vi "Page_Advanced_WriteAll.vi"(6 "ctl references":T1, 8 "error in (no error)":errorcluster, 11 "AB_Application in":refnum<class "AB_Application.lvclass">) -> (0 "error out":errorcluster, 3 "AB_Application out":refnum<class "AB_Application.lvclass">)   [LabVIEW 2020, in "AB_Application.lvclass"]
uses:
  <vilib>/AppBuilder/AB_Classes/Application/AB_Application.lvclass
  <vilib>/AppBuilder/AB_Classes/Application/AB_Application.lvclass/AB_Application.ctl
  <vilib>/AppBuilder/AB_Classes/TargetFile/AB_Targetfile.lvclass
  <resource>/Framework/Providers/Builds/AppBuilder/AB_UI_Page_Advanced_References.ctl
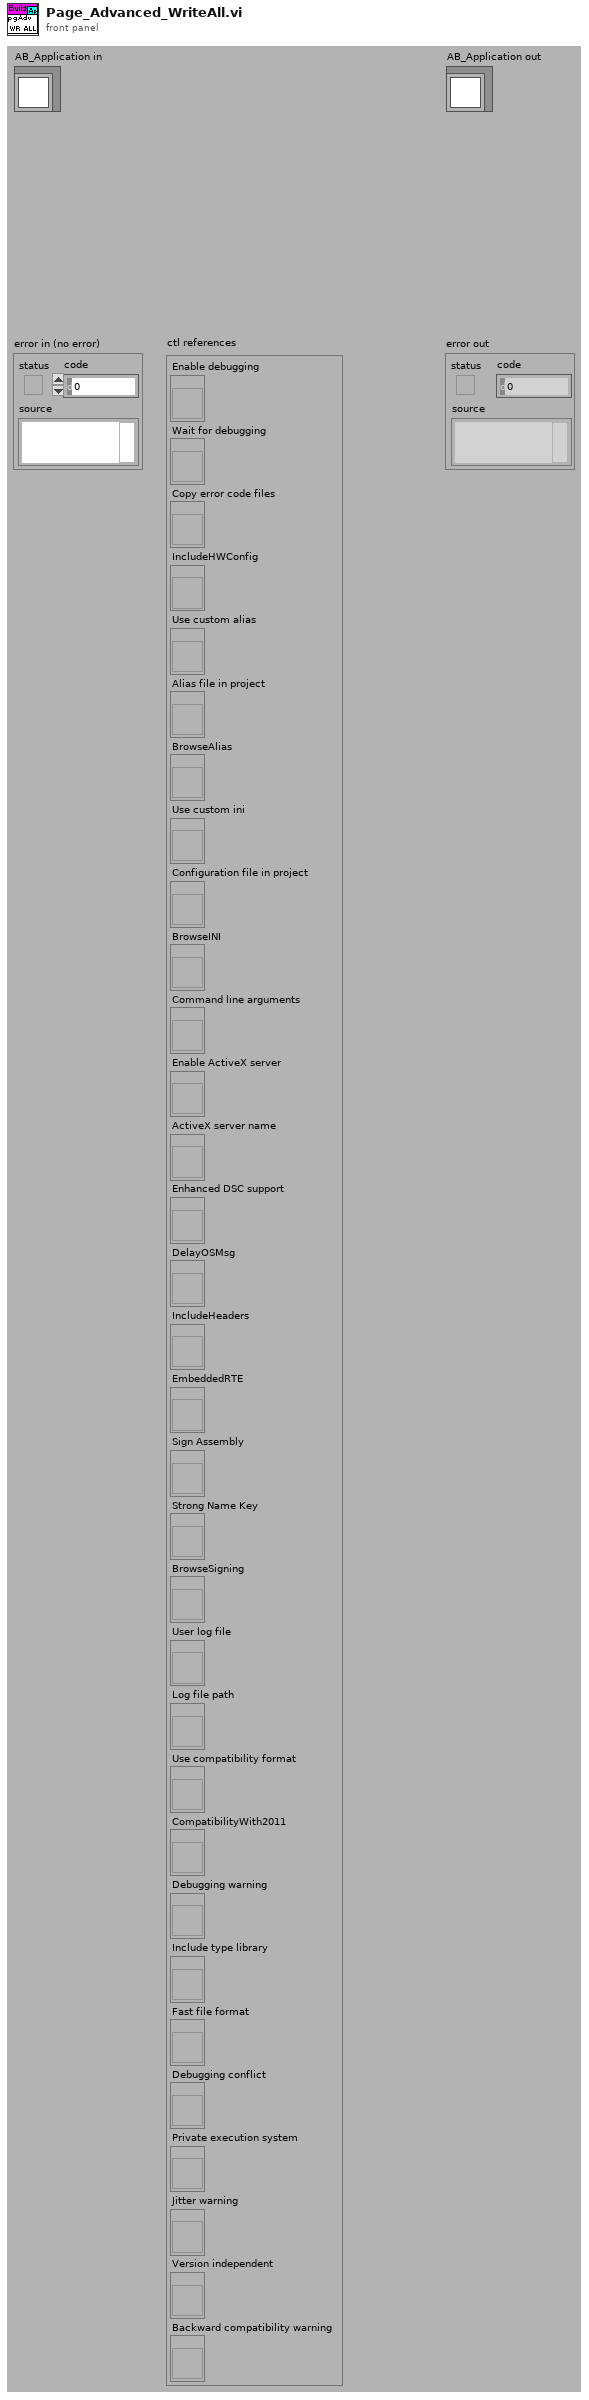
[diagram p1: front panel]
types:
  T1 = typedef "AB_UI_Page_Advanced_References.ctl" = cluster{"Enable debugging":refnum<vi>, "Wait for debugging":refnum<vi>, "Copy error code files":refnum<vi>, "IncludeHWConfig":refnum<vi>, "Use custom alias":refnum<vi>, "Alias file in project":refnum<vi>, "BrowseAlias":refnum<vi>, "Use custom ini":refnum<vi>, "Configuration file in project":refnum<vi>, "BrowseINI":refnum<vi>, "Command line arguments":refnum<vi>, "Enable ActiveX server":refnum<vi>, "ActiveX server name":refnum<vi>, "Enhanced DSC support":refnum<vi>, "DelayOSMsg":refnum<vi>, "IncludeHeaders":refnum<vi>, "EmbeddedRTE":refnum<vi>, "Sign Assembly":refnum<vi>, "Strong Name Key":refnum<vi>, "BrowseSigning":refnum<vi>, "User log file":refnum<vi>, "Log file path":refnum<vi>, "Use compatibility format":refnum<vi>, "CompatibilityWith2011":refnum<vi>, "Debugging warning":refnum<vi>, "Include type library":refnum<vi>, "Fast file format":refnum<vi>, "Debugging conflict":refnum<vi>, "Private execution system":refnum<vi>, "Jitter warning":refnum<vi>, "Version independent":refnum<vi>, "Backward compatibility warning":refnum<vi>}
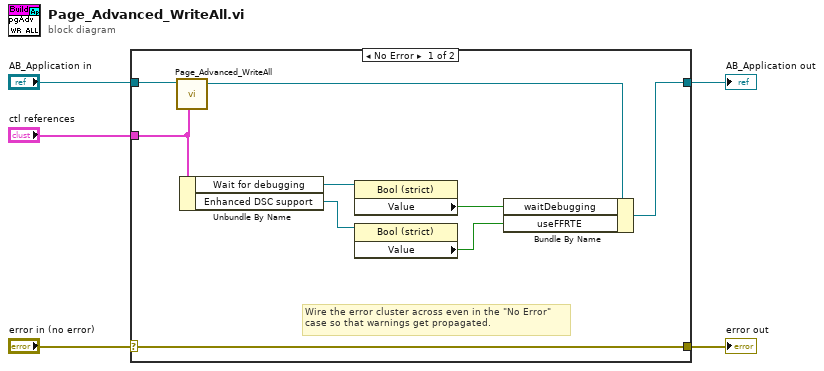
[diagram p0: block diagram]
diagram:
  n1 = case shown="No Error" "error in (no error)" {
    selector: "error in (no error)" -> [w14 w16]
    tunnel: [w14 w16] -> w4
    tunnel: [w13 w15] -> w2
    tunnel: "AB_Application in" -> [w8 w15]
    tunnel: "ctl references" -> [w7 _]
    frame No Error {
      # "Wire the error cluster across even in the \"No Error\"\ncase so that warnings get propagated."
      n2 = call-parent "Page_Advanced_WriteAll.vi"("ctl references"=w7, "AB_Targetfile in"=w8) -> ("AB_Targetfile out"=w6:refnum<class "AB_Application.lvclass">)  [unwired: 1 in, 8 out]
      n3 = Unbundle By Name(w7) -> ("Wait for debugging"=w12:refnum<vi>, "Enhanced DSC support"=w10:refnum<vi>)
      n4 = property class="Bool (strict)"(reference=w12) -> ("Value"=w11:bool)  [unwired: 1 in, 2 out]
      n5 = property class="Bool (strict)"(reference=w10) -> ("Value"=w9:bool)  [unwired: 1 in, 2 out]
      n6 = Bundle By Name(cluster=w6, "waitDebugging"=w11, "useFFRTE"=w9) -> (w13:refnum<class "AB_Application.lvclass">)
    }
    frame Error {
    }
  }
  "error out" <- w4
  "AB_Application out" <- w2
